vi "秒转分.vi"(3 "秒计数":dbl) -> (1 "分钟数":string)   [LabVIEW 2014]
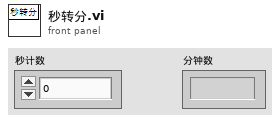
[diagram p1: front panel]
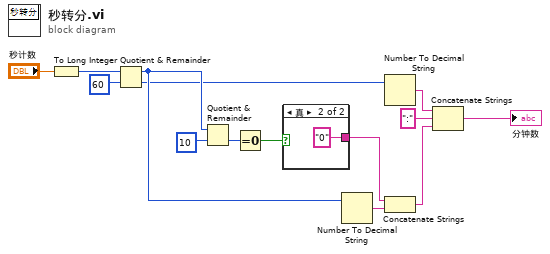
[diagram p0: block diagram]
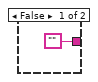
[diagram p2: hidden frame]
diagram:
  n1 = To Long Integer(number="秒计数") -> (32bit integer=w14:i32)
  n2 = Quotient & Remainder(x=w14, y=60) -> (x-y*floor(x/y)=w8:i32, floor(x/y)=w1:i32)
  n3 = Quotient & Remainder(x=w8, y=10) -> (floor(x/y)=w7:i32)  [unwired: 1 out]
  n4 = Equal To 0?(x=w7) -> (x = 0?=w12:bool)
  n5 = case shown="真" w12 {
    tunnel: ["" "0"] -> w11
    frame False {
    }
    frame True {
    }
  }
  n6 = Number To Decimal String(number=w8) -> (decimal integer string=w10:string)  [unwired: 1 in]
  n7 = Number To Decimal String(number=w1) -> (decimal integer string=w6:string)  [unwired: 1 in]
  n8 = Concatenate Strings(w11, w10) -> (w4:string)
  n9 = Concatenate Strings(w6, ":", w4) -> (→"分钟数":string)
